vi "XML429_Channel_GetChannelDirection.vi"(0 "Channel in":refnum<k20>, 11 "Error in":errorcluster) -> (4 "Channel out":refnum<k20>, 6 "ChannelDirection":T1(ring), 15 "Error out":errorcluster)   [LabVIEW 2016]
doc: "XML429_Channel_GetChannelDirection"
uses:
  <vilib>/Utility/error.llb/Error Cluster From Error Code.vi
  <vilib>/xml/Close Reference(Node).vi
  <vilib>/ErrorRing/Error Ring.xnode
  <vilib>/xml/NI_XML.lvlib
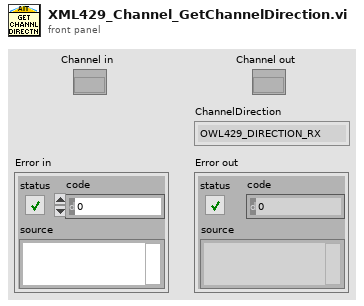
[diagram p1: front panel]
types:
  T1 = enum16{"OWL429_DIRECTION_RX", "OWL429_DIRECTION_TX"}
  T2 = enum16{"OWL429_DIRECTION_RX", "OWL429_DIRECTION_TX"}[]
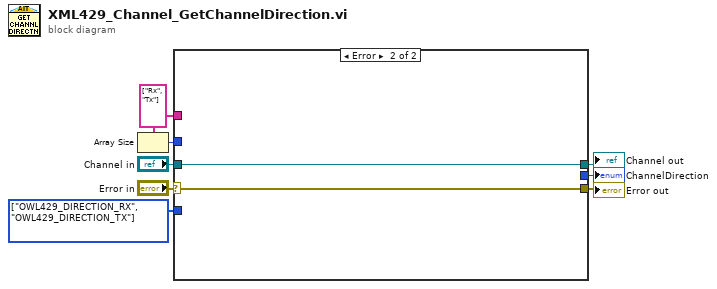
[diagram p0: block diagram]
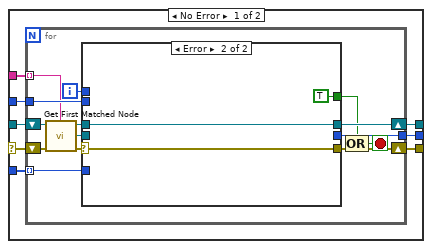
[diagram p2: hidden frame]
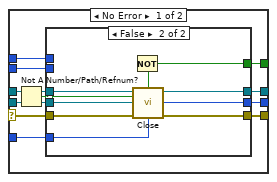
[diagram p3: hidden frame]
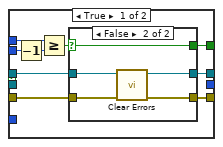
[diagram p4: hidden frame]
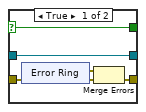
[diagram p5: hidden frame]
diagram:
  w2 = T2 [enum."OWL429_DIRECTION_RX", enum."OWL429_DIRECTION_TX"] items=["OWL429_DIRECTION_RX", "OWL429_DIRECTION_TX"]
  w4 = string[] ["Rx", "Tx"]
  n1 = Array Size(array=w4) -> (size(s)=w3:i32)
  n2 = case shown="Error" "Error in" {
    selector: "Error in" -> [w15 w75]
    tunnel: [w16 w75] -> w7
    tunnel: "Channel in" -> [w13 w74]
    tunnel: [w14 w74] -> w5
    tunnel: w4 -> [w10 _]
    tunnel: w3 -> [w12 _]
    tunnel: [w11 _] -> w1
    tunnel: w2 -> [w9 _]
    frame No Error {
      n3 = for {
        shift-right: [w20] -> w16
        shift-left: w15 -> [w29]
        shift-right: [w26] -> w14
        shift-left: w13 -> [w30]
        tunnel: w12 -> [w23]
        tunnel: [w22] -> w11
        tunnel: w10 -> [w21] mode=indexing
        tunnel: w9 -> [w17] mode=indexing
        i -> [w24]
        stop <- w18 stop-if-true
        n4 = call <vilib>:"Get First Matched Node.vi"("error in (no error)"=w29, "XPath expression"=w21, "node in"=w30) -> ("error out"=w28:errorcluster, "node result"=w25:refnum<k20>, "node out"=w27:refnum<k20>)  [unwired: 6 in]
        n5 = case shown="Error" w28 {
          selector: w28 -> [w41 w73]
          tunnel: [w40 w73] -> w20
          tunnel: [w38 w72] -> w26
          tunnel: w27 -> [w39 w72]
          tunnel: w25 -> [w34 _]
          tunnel: w24 -> [w36 _]
          tunnel: w23 -> [w35 _]
          tunnel: [w33 TRUE] -> w19
          tunnel: [w32 _] -> w22
          tunnel: w17 -> [w31 _]
          frame No Error {
            n6 = Not A Number/Path/Refnum?(number/path/refnum=w34) -> (NaN/Path/Refnum?=w37:bool)
            n7 = case shown="False" w37 {
              selector: w37 -> [_ w69]
              tunnel: [w49 w65] -> w40
              tunnel: w41 -> [w50 w66]
              tunnel: [w43 w70] -> w38
              tunnel: w39 -> [w44 w70]
              tunnel: w36 -> [w47 _]
              tunnel: w35 -> [w48 _]
              tunnel: w34 -> [_ w64]
              tunnel: [w42 w68] -> w33
              tunnel: [_ w67] -> w32
              tunnel: w31 -> [_ w67]
              frame True {
                n8 = Decrement(x=w48) -> (x-1=w46:i32)
                n9 = Greater Or Equal?(x=w47, y=w46) -> (x >= y?=w45:bool)
                n10 = case shown="False" w45 {
                  selector: w45 -> [w51 w60]
                  tunnel: w50 -> [w53 w63]
                  tunnel: [w54 w62] -> w49
                  tunnel: [w55 w61] -> w43
                  tunnel: w44 -> [w55 w61]
                  tunnel: [w51 w60] -> w42
                  frame True {
                    n11 = xnode "Error Ring"() -> ("error out"=w52:errorcluster)
                    n12 = Merge Errors(w53, w52) -> (w54:errorcluster)
                  }
                  frame False, Default {
                    n13 = call <vilib>:"Clear Errors.vi"("error in (no error)"=w63) -> ("error out"=w62:errorcluster)  [unwired: 5 in, 1 out]
                  }
                }
              }
              frame False, Default {
                n14 = Not(x=w69) -> (.not. x?=w68:bool)
                n15 = call-poly <vilib>:"Close.vi"("error in (no error)"=w66, "node"=w64) -> ("error out"=w65:errorcluster)  [unwired: 7 in]
              }
            }
          }
          frame Error {
          }
        }
        n16 = Compound Arithmetic op=OR(w19, w20) -> (w18:bool)
      }
    }
    frame Error {
    }
  }
  "Error out" <- w7
  "Channel out" <- w5
  "ChannelDirection" <- w1
